vi "Console - Show Front Panel (Read-Only).vi"(11 "Display Console":bool) -> ()   [LabVIEW 2017, in "Communications Console Library.lvlib"]
uses:
  Communications Console Library.lvlib
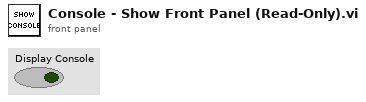
[diagram p1: front panel]
types:
  T1 = enum32{"Invalid", "Standard", "Closed", "Hidden", "Minimized", "Maximized"}
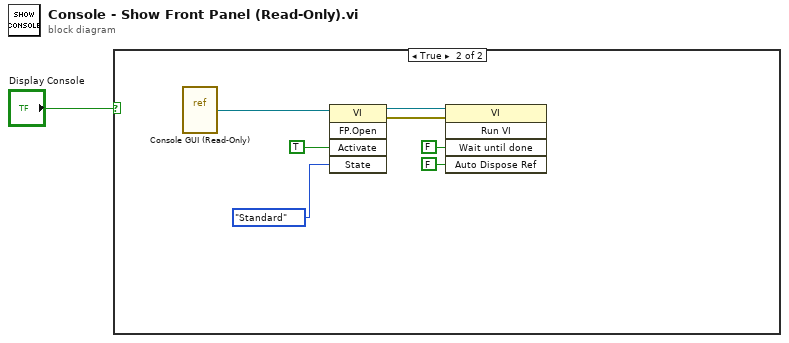
[diagram p0: block diagram]
diagram:
  n1 = case shown="True" "Display Console" {
    frame False {
    }
    frame True {
      n2 = vi-ref "Console GUI (Read-Only).vi"() -> (w8:refnum<vi>)
      n3 = invoke class="VI" method="FP.Open"(reference=w8, "Activate"=TRUE ("Activate?"), "State"=T1."Standard") -> (reference out=w5:refnum<vi>, error out=w4:errorcluster)  [unwired: 2 in, 3 out]
      n4 = invoke class="VI" method="Run VI"(reference=w5, error in=w4, "Wait until done"=FALSE ("Wait Until Done"), "Auto Dispose Ref"=FALSE ("Auto Dispose Reference")) -> ()  [unwired: 1 in, 5 out]
    }
  }
